vi "Prepare Test.vi"(8 "error in (no error)":errorcluster, 11 "LVUnit Test Case.lvclass":refnum<class "LVUnit Test Case.lvclass">) -> (0 "error out":errorcluster, 2 "VI Refnum":refnum<vi>)   [LabVIEW 2017, in "LVUnit Test Executor.lvclass"]
doc: "Prepares the specified test case for execution."
uses:
  LVUnit Test Executor.lvclass
  LVUnit Test Case/LVUnit Test Case.lvclass
  C:/Users/pasca/source/repos/lvunit/Test Case/Test Case.lvclass
  Test Case/Test Case.lvclass/Test Case.ctl
  LVUnit Test Case/LVUnit Test Case.lvclass/LVUnit Test Case.ctl
  <vilib>/PNR/JSONtext Object Serialization/Generic Object Serializer/Generic Object Serializer.lvclass
  C:/Program Files (x86)/National Instruments/LabVIEW 2017/vi.lib/JDP Science/JSONtext/LVClass Serializer/JSONtext LVClass Serializer.lvclass
  <vilib>/PNR/JSONtext Object Serialization/Generic Object Serializer/Type Name Handling.ctl
  <vilib>/PNR/JSONtext Object Serialization/Generic Object Serializer/Generic Object Serializer.lvclass/Generic Object Serializer.ctl
  bede4881-c3ee-429c-a29f-335cd5e8a060.vi
  <vilib>/PNR/JSONtext Object Serialization/Generic Object Serializer/Write Type Name Handling.vi
  Test Case/Get Path.vi
  LVUnit Test Case/Get JSON Data.vi
  <vilib>/JDP Science/JSONtext/Find Item.vi
  <vilib>/JDP Science/JSONtext/String Subset.vi
  <vilib>/JDP Science/JSONtext/Parsing/Parse Full Path or Item Name.vi
  <vilib>/JDP Science/JSONtext/Next JSON Value.vi
  <vilib>/JDP Science/JSONtext/support/Error Cluster From Code.vi
  <vilib>/JDP Science/JSONtext/Offset/Find Item Locations by Path.vi
  <vilib>/JDP Science/JSONtext/JSON text to Variant.vi
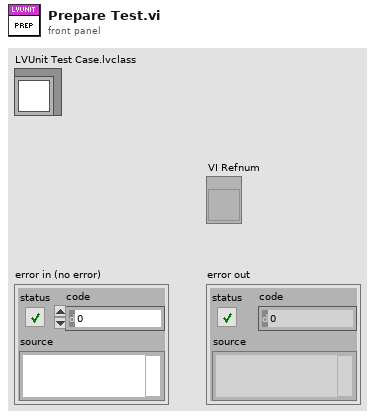
[diagram p1: front panel]
types:
  T1 = typedef "Generic Object Serializer.lvclass/Type Name Handling.ctl" = enum16{"None", "Inline"}
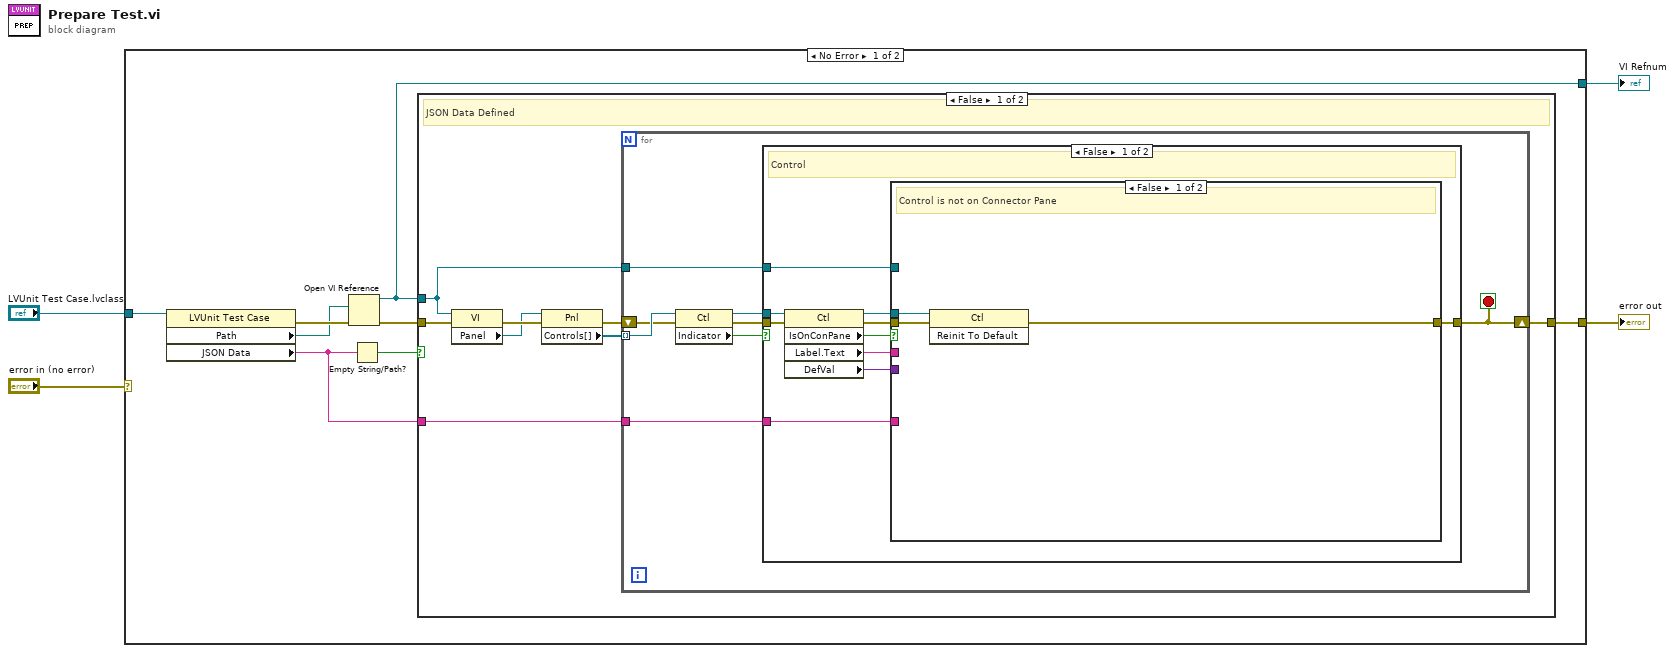
[diagram p0: block diagram]
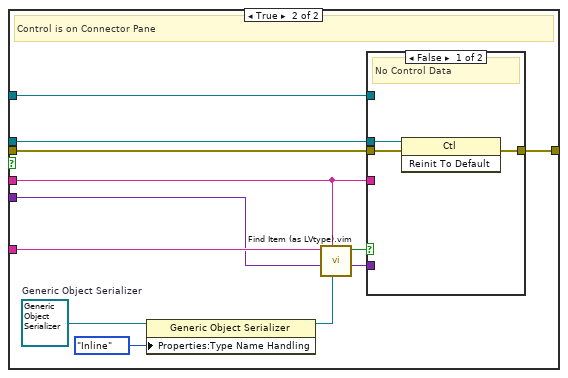
[diagram p2: hidden frame]
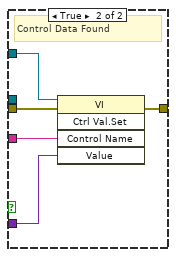
[diagram p3: hidden frame]
diagram:
  n1 = case shown="No Error" "error in (no error)" {
    selector: "error in (no error)" -> [_ w64]
    tunnel: [w9 _] -> w4
    tunnel: "LVUnit Test Case.lvclass" -> [w8 _]
    tunnel: [w7 w64] -> w2
    frame No Error {
      n2 = property class="LVUnit Test Case"(reference=w8) -> (error out=w12:errorcluster, "Path"=w11:path, "JSON Data"=w5:string)  [unwired: 1 in, 1 out]
      n3 = Open VI Reference(vi path=w11, error in (no error)=w12) -> (vi reference=w9:refnum<vi>, error out=w10:errorcluster)  [unwired: 4 in]
      n4 = Empty String/Path?(string/path=w5) -> (empty?=w6:bool)
      n5 = case shown="False" w6 {
        tunnel: w10 -> [w20 w63]
        tunnel: [w19 w63] -> w7
        tunnel: w9 -> [w18 _]
        tunnel: w5 -> [w17 _]
        frame False {
          # "JSON Data Defined"
          n6 = property class="VI"(reference=w18, error in=w20) -> (error out=w16:errorcluster, "Panel"=w14:refnum<vi>)  [unwired: 1 out]
          n7 = property class="Pnl"(reference=w14, error in=w16) -> (error out=w15:errorcluster, "Controls[]"=w13:refnum<vi>[])  [unwired: 1 out]
          n8 = for {
            tunnel: w18 -> [w27]
            shift-right: [w26] -> w19
            shift-left: w15 -> [w24]
            tunnel: w17 -> [w28]
            tunnel: w13 -> [w25] mode=indexing
            stop <- w26 stop-if-true
            n9 = property class="Ctl"(reference=w25, error in=w24) -> (reference out=w23:refnum<vi>, error out=w22:errorcluster, "Indicator"=w21:bool)
            n10 = case shown="False" w21 {
              tunnel: w28 -> [w36 _]
              tunnel: w27 -> [w33 _]
              tunnel: [w32 w62] -> w26
              tunnel: w23 -> [w31 _]
              tunnel: w22 -> [w30 w62]
              frame False {
                # "Control"
                n11 = property class="Ctl"(reference=w31, error in=w30) -> (reference out=w34:refnum<vi>, error out=w37:errorcluster, "IsOnConPane"=w38:bool, "Label.Text"=w35:string, "DefVal"=w29:variant)
                n12 = case shown="False" w38 {
                  tunnel: [w40 w51] -> w32
                  tunnel: w37 -> [w41 w53]
                  tunnel: w36 -> [_ w50]
                  tunnel: w35 -> [_ w42]
                  tunnel: w34 -> [w39 w46]
                  tunnel: w33 -> [_ w52]
                  tunnel: w29 -> [_ w49]
                  frame False {
                    # "Control is not on Connector Pane"
                    n13 = invoke class="Ctl" method="Reinit To Default"(reference=w39, error in=w41) -> (error out=w40:errorcluster)  [unwired: 1 in, 2 out]
                  }
                  frame True {
                    w45 = refnum<class "Generic Object Serializer.lvclass"> refnum  # Generic Object Serializer
                    # "Control is on Connector Pane"
                    n14 = property class="Generic Object Serializer"(reference=w45, "Properties:Type Name Handling"=Type_Name_Handling."Inline" ("Type Name Handling")) -> (reference out=w44:refnum<class "Generic Object Serializer.lvclass">)  [unwired: 1 in, 1 out]
                    n15 = call "Find Item (as LVtype).vim"("LVClass Serializer"=w44, "$Path or Item Name"=w42, "Data Type and Default Value"=w49, "JSON"=w50) -> ("Data"=w48:variant, "Found"=w47:bool)  [unwired: 4 in, 2 out]
                    n16 = case shown="False" w47 {
                      tunnel: w53 -> [w56 w61]
                      tunnel: w52 -> [_ w60]
                      tunnel: [w55 w59] -> w51
                      tunnel: w42 -> [_ w58]
                      tunnel: w48 -> [_ w57]
                      tunnel: w46 -> [w54 _]
                      frame False {
                        # "No Control Data"
                        n17 = invoke class="Ctl" method="Reinit To Default"(reference=w54, error in=w56) -> (error out=w55:errorcluster)  [unwired: 1 in, 2 out]
                      }
                      frame True {
                        # "Control Data Found"
                        n18 = invoke class="VI" method="Ctrl Val.Set"(reference=w60, error in=w61, "Control Name"=w58, "Value"=w57) -> (error out=w59:errorcluster)  [unwired: 1 in, 4 out]
                      }
                    }
                  }
                }
              }
              frame True {
                # "Indicator"
              }
            }
          }
        }
        frame True {
          # "No JSON Data"
        }
      }
    }
    frame Error {
    }
  }
  "VI Refnum" <- w4
  "error out" <- w2
